vi "624_Get All Control References.vi"(8 "error in (no error)":errorcluster, 11 "Controls[] in":refnum<vi>[](array[refnum])) -> (0 "error out":errorcluster, 2 "Warnings List":string, 3 "Named Controls":T1)   [LabVIEW 2013]
doc: "The Get All Control References VI recursively determines control references for all objects on the front panel of another VI. This VI takes a front panel reference input and returns an array of references to all controls on that front panel. This VI returns references to all elements of a cluster, including elements in embedded clusters. This VI also returns the element types of arrays embedded in cluster elements."
uses:
  Named Control.ctl
panel:
  in  "target class 2":refnum<vi>
  in  "target class":refnum<vi>
  # "Select Help»Show Context Help and move the cursor over the VI icon to display help for this VI."
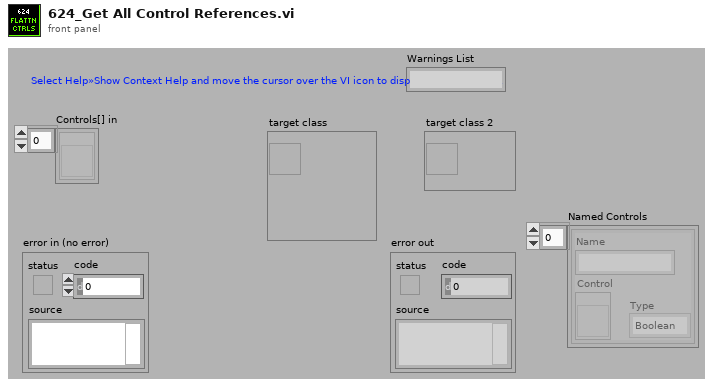
[diagram p1: front panel]
types:
  T1 = typedef "Named Control.ctl" = cluster{"Name":string, "Control":refnum<vi>, "Type":enum16{"Boolean", "Double"}}[]
  T2 = cluster{"Name":string, "Control":refnum<vi>, "Type":enum16{"Boolean", "Double"}}
  T3 = typedef "Field Data.ctl" = cluster{"Dbl":dbl, "String":string, "Type":T4, "Boolean":bool, "Sequence #":T5}
  T4 = typedef "Field Type.ctl" = enum8{"Invalid", "Bool", "Numeric", "String", "Boolean Array", "Numeric Array", "String Array"}
  T5 = typedef "Sequence.ctl" = u16
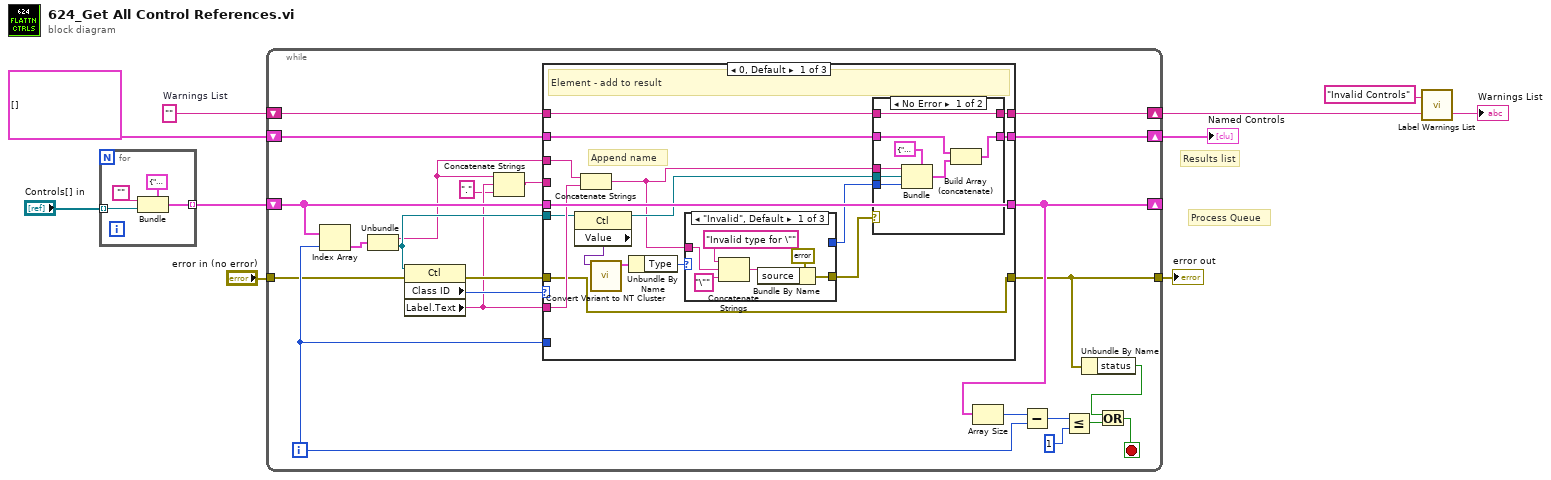
[diagram p0: block diagram]
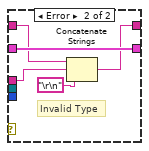
[diagram p2: hidden frame]
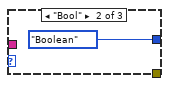
[diagram p3: hidden frame]
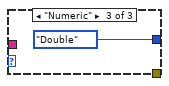
[diagram p4: hidden frame]
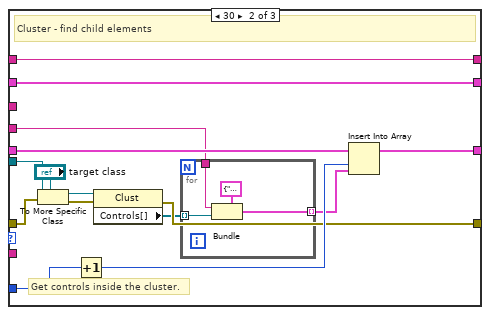
[diagram p5: hidden frame]
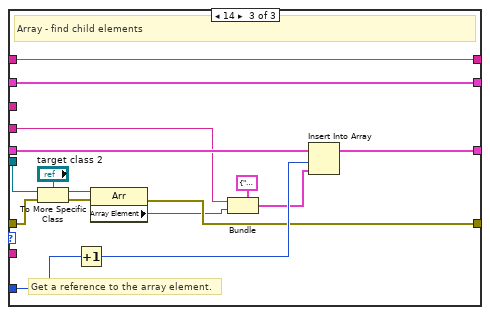
[diagram p6: hidden frame]
diagram:
  w4 = ""  # Warnings List
  # "Results list"
  # "Process Queue"
  n1 = for {
    tunnel: "Controls[] in" -> [w13] mode=indexing
    tunnel: [w12] -> w7 mode=indexing
    n2 = Bundle(cluster=cluster{"String":string, "element":refnum<vi>} {"String"="", "element"=refnum} ("Named Controls"), "String"="", "element"=w13) -> (w12:cluster{"String":string, "element":refnum<vi>})
  }
  n3 = while {
    shift-right: [w30] -> _
    shift-left: w7 -> [w25]
    tunnel: "error in (no error)" -> [w29]
    tunnel: [w26] -> w10
    shift-right: [w23] -> w6
    shift-left: T1 [] ("Named Controls 2") -> [w24]
    shift-right: [w15] -> w3
    shift-left: w4 -> [w16]
    i -> [w34]
    stop <- w32 stop-if-true
    n4 = Index Array(array=w25, index=w34) -> (element=w22:cluster{"String":string, "element":refnum<vi>})
    n5 = Unbundle(w22) -> ("String"=w20:string, "element"=w21:refnum<vi>)
    n6 = property class="Ctl"(reference=w21, error in=w29) -> (error out=w28:errorcluster, "Class ID"=w31:u32, "Label.Text"=w19:string)  [unwired: 1 out]
    n7 = Concatenate Strings(w20, w19, "." ("string")) -> (w17:string)
    n8 = case shown="0, Default" w31 {
      tunnel: w25 -> [w53 w87 w107]
      tunnel: w34 -> [_ w86 w106]
      tunnel: [w53 w85 w105] -> w30
      tunnel: w28 -> [w40 w83 w103]
      tunnel: [w40 w81 w101] -> w26
      tunnel: w24 -> [w52 w80 w100]
      tunnel: [w51 w80 w100] -> w23
      tunnel: w21 -> [w48 w79 w95]
      tunnel: w20 -> [w50 _ _]
      tunnel: w19 -> [w49 _ _]
      tunnel: w17 -> [_ w76 w97]
      tunnel: w16 -> [w39 w75 w94]
      tunnel: [w38 w75 w94] -> w15
      frame 0, Default {
        # "Append name"
        # "Element - add to result"
        n9 = property class="Ctl"(reference=w48) -> (reference out=w47:refnum<vi>, "Value"=w46:variant)  [unwired: 1 in, 1 out]
        n10 = Concatenate Strings(w50, w49) -> (w42:string)
        n11 = call <vilib>:"Convert Variant to NT Cluster.vi"("NewVal"=w46) -> ("Field Value"=w45:T3)  [unwired: 10 in]
        n12 = Unbundle By Name(w45) -> ("Type"=w44:T4)
        n13 = case shown="\"Invalid\", Default" w44 {
          tunnel: [_ enum16{"Boolean", "Double"}."Boolean" ("Type") enum16{"Boolean", "Double"}."Double" ("Type")] -> w43
          tunnel: [w68 _ _] -> w41
          tunnel: w42 -> [w67 _ _]
          frame "Invalid", Default {
            n14 = Concatenate Strings("Invalid type for \"" ("string"), w67, "\"" ("string")) -> (w70:string)
            n15 = Bundle By Name(cluster=errorcluster {"status"=TRUE, "code"=1, "source"=""} ("error out"), "source"=w70) -> (w68:errorcluster)
          }
          frame "Bool" {
          }
          frame "Numeric" {
          }
        }
        n16 = case shown="No Error" w41 {
          tunnel: w52 -> [w61 w66]
          tunnel: [w60 w66] -> w51
          tunnel: w47 -> [w58 _]
          tunnel: w43 -> [w57 _]
          tunnel: w42 -> [w55 w63]
          tunnel: w39 -> [w54 w65]
          tunnel: [w54 w64] -> w38
          frame No Error {
            n17 = Bundle(cluster=T2 {"Name"="", "Control"=refnum, "Type"=enum."Boolean"} ("Named Controls"), "Name"=w55, "Control"=w58, "Type"=w57) -> (w56:T2)
            n18 = Build Array (concatenate)(w61, w56) -> (w60:T1)
          }
          frame Error {
            # "Invalid Type"
            n19 = Concatenate Strings(w65, w63, "\r\n") -> (w64:string)
          }
        }
      }
      frame 30 {
        # "Get controls inside the cluster."
        # "Cluster - find child elements"
        n20 = To More Specific Class(target class="target class", reference=w79, error in=w83) -> (specific class reference=w89:refnum<vi>, error out=w82:errorcluster)
        n21 = Increment(x=w86) -> (x+1=w84:i32)
        n22 = property class="Clust"(reference=w89, error in=w82) -> (error out=w81:errorcluster, "Controls[]"=w78:refnum<vi>[])  [unwired: 1 out]
        n23 = for {
          tunnel: w78 -> [w92] mode=indexing
          tunnel: w76 -> [w91]
          tunnel: [w90] -> w77 mode=indexing
          n24 = Bundle(cluster=cluster{"String":string, "element":refnum<vi>} {"String"="", "element"=refnum} ("Named Controls"), "String"=w91, "element"=w92) -> (w90:cluster{"String":string, "element":refnum<vi>})
        }
        n25 = Insert Into Array(array=w87, index=w84, new element=w77) -> (w85:cluster{"String":string, "element":refnum<vi>}[])
      }
      frame 14 {
        # "Get a reference to the array element."
        # "Array - find child elements"
        n26 = To More Specific Class(target class="target class 2", reference=w95, error in=w103) -> (specific class reference=w109:refnum<vi>, error out=w102:errorcluster)
        n27 = Increment(x=w106) -> (x+1=w104:i32)
        n28 = property class="Arr"(reference=w109, error in=w102) -> (error out=w101:errorcluster, "Array Element"=w98:refnum<vi>)  [unwired: 1 out]
        n29 = Bundle(cluster=cluster{"String":string, "element":refnum<vi>} {"String"="", "element"=refnum} ("Named Controls"), "String"=w97, "element"=w98) -> (w96:cluster{"String":string, "element":refnum<vi>})
        n30 = Insert Into Array(array=w107, index=w104, new element=w96) -> (w105:cluster{"String":string, "element":refnum<vi>}[])
      }
    }
    n31 = Array Size(array=w30) -> (size(s)=w37:i32)
    n32 = Subtract(x=w37, y=w34) -> (x-y=w36:i32)
    n33 = Less Or Equal?(x=w36, y=1) -> (x <= y?=w33:bool)
    n34 = Unbundle By Name(w26) -> ("status"=w27:bool)
    n35 = Or(x=w27, y=w33) -> (x .or. y?=w32:bool)
  }
  "error out" <- w10
  "Named Controls" <- w6
  n36 = call "Label Warnings List.vi"("Warnings List in"=w3, "Section"="Invalid Controls") -> ("Warnings List out"=→"Warnings List":string)  [unwired: 1 in]
